vi "scale.vi"() -> (3 "Game Specific Data":string)   [LabVIEW 2017]
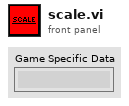
[diagram p1: front panel]
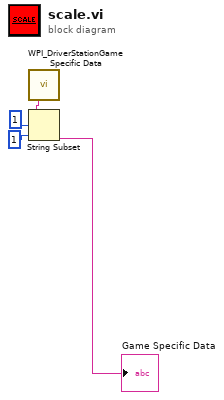
[diagram p0: block diagram]
diagram:
  n1 = call <vilib>:"WPI_DriverStationGame Specific Data.vi"() -> ("Game Specific Data"=w4:string)  [unwired: 11 in]
  n2 = String Subset(string=w4, offset (0)=1, length (rest)=1 ("length (rest)")) -> (substring=→"Game Specific Data":string)
